vi "Register Data Emitters.vi"(8 "error in (no error)":errorcluster, 10 "Emitter":string, 11 "gController in":refnum<class "gController.lvclass">) -> (0 "error out":errorcluster, 3 "gController out":refnum<class "gController.lvclass">)   [LabVIEW 2016, in "Controller.lvlib" / "gController.lvclass"]
uses:
  gController.lvclass
  gController.lvclass/gController.ctl
  <vilib>/MSR Consulting, LLC/General Reuse/Data/Data.lvclass
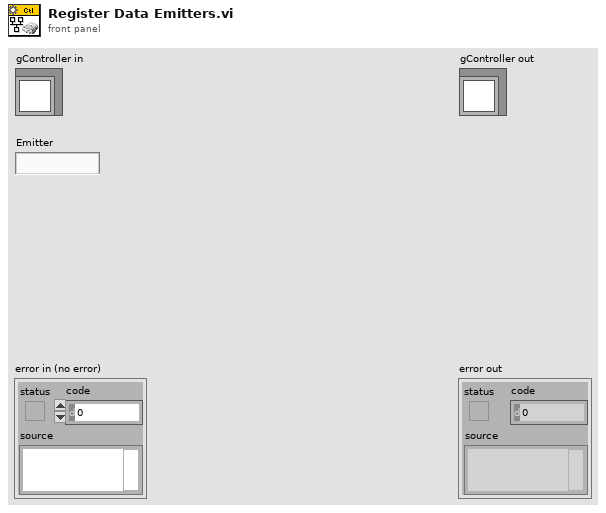
[diagram p1: front panel]
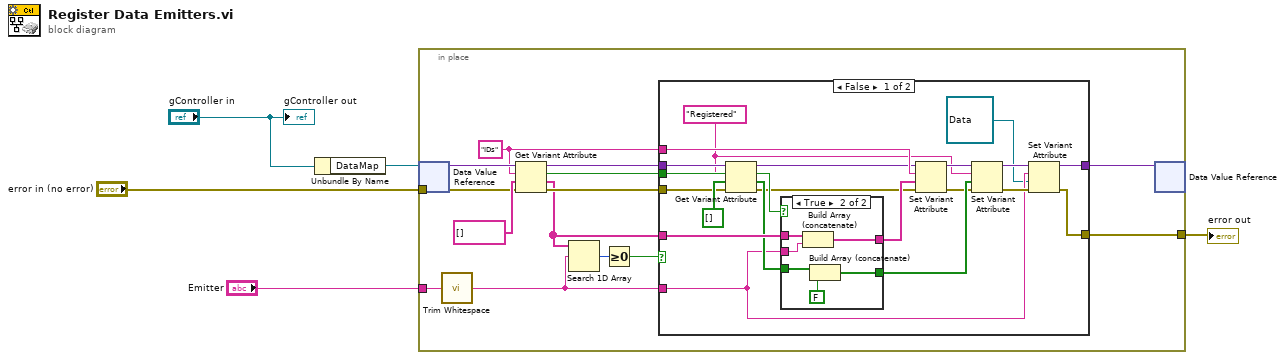
[diagram p0: block diagram]
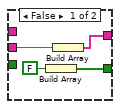
[diagram p2: hidden frame]
diagram:
  n1 = Unbundle By Name("gController in") -> ("DataMap"=w5:refnum<data-value>)
  n2 = in-place {
    in-place-border: "Emitter" -> [w10]
    in-place-border: "error in (no error)" -> [w13]
    in-place-border: [w11] -> w2
    w16 = "IDs" ("name")
    n3 = in-place-dvr #1(w5) -> (w19:variant)  [unwired: 1 out]
    n4 = call <vilib>:"Trim Whitespace.vi"("string"=w10) -> ("trimmed string"=w8:string)  [unwired: 1 in]
    n5 = Get Variant Attribute(Variant=w19, name=w16, default value (empty Variant)=string[] [], error in=w13) -> (duplicate Variant=w15:variant, found=w17:bool, value=w9:string[], error out=w14:errorcluster)
    n6 = Search 1D Array(1D array=w9, element=w8) -> (index of element=w7:i32)  [unwired: 1 in]
    n7 = Greater Or Equal To 0?(x=w7) -> (x >= 0?=w6:bool)
    n8 = case shown="False" w6 {
      tunnel: w17 -> [w39 _]
      tunnel: w9 -> [w38 _]
      tunnel: w16 -> [w37 _]
      tunnel: w15 -> [w34 w51]
      tunnel: w14 -> [w26 w50]
      tunnel: [w23 w51] -> w12
      tunnel: [w22 w50] -> w11
      tunnel: w8 -> [w21 _]
      frame False {
        w29 = "Registered" ("name")
        n9 = Get Variant Attribute(Variant=w34, name=w29, default value (empty Variant)=bool[] [], error in=w26) -> (duplicate Variant=w33:variant, value=w32:bool[], error out=w27:errorcluster)  [unwired: 1 out]
        n10 = case shown="True" w39 {
          tunnel: w38 -> [_ w49]
          tunnel: w21 -> [w43 w48]
          tunnel: [w42 w47] -> w36
          tunnel: w32 -> [_ w46]
          tunnel: [w40 w45] -> w31
          frame False {
            n11 = Build Array(FALSE) -> (w40:bool[])
            n12 = Build Array(w43) -> (w42:string[])
          }
          frame True {
            n13 = Build Array (concatenate)(w49, w48) -> (w47:string[])
            n14 = Build Array (concatenate)(w46, FALSE) -> (w45:bool[])
          }
        }
        n15 = Set Variant Attribute(Variant=w33, name=w37, value=w36, error in=w27) -> (Variant out=w30:variant, error out=w28:errorcluster)  [unwired: 1 out]
        n16 = Set Variant Attribute(Variant=w30, name=w29, value=w31, error in=w28) -> (Variant out=w25:variant, error out=w24:errorcluster)  [unwired: 1 out]
        n17 = Set Variant Attribute(Variant=w25, name=w21, value=refnum<class "Data.lvclass"> refnum ("Base Data Lib:Data"), error in=w24) -> (Variant out=w23:variant, error out=w22:errorcluster)  [unwired: 1 out]
      }
      frame True {
        # "Emitters can already be registered if an actor is launched and returning data before this is run.  Prevent multiple registration..."
      }
    }
    n18 = in-place-dvr #1(w12) -> ()  [unwired: 2 out]
  }
  "error out" <- w2
  "gController out" <- "gController in"
